vi "Get JSON Data.vi"(7 "Panel Origin":T1, 8 "error in (no error)":errorcluster, 9 "Force Get All Data":bool, 10 "VI Reference":refnum<vi>, 11 "Text In":refnum<class "Text.lvclass">) -> (0 "error out":errorcluster, 2 "JSON string":string, 3 "Text Out":refnum<class "Text.lvclass">)   [LabVIEW 2015, in "Front Panel Publisher.lvlib" / "Text.lvclass"]
uses:
  Text.lvclass
  <vilib>/Utility/miscctls.llb/LVPointTypeDef.ctl
  Object_class/Object.lvclass
  Web Front Panel_class/Web Front Panel.lvclass
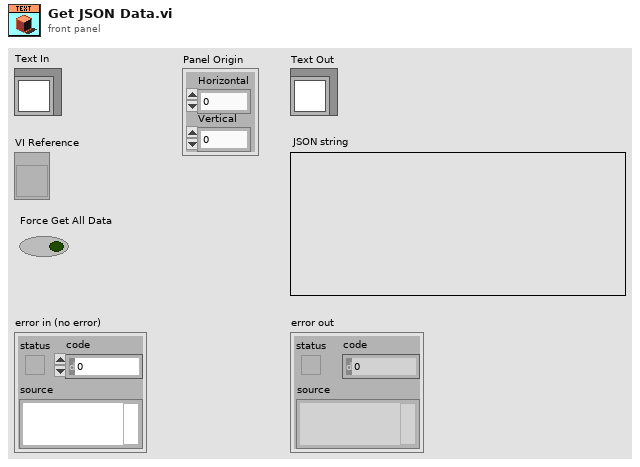
[diagram p1: front panel]
types:
  T1 = typedef "LVPointTypeDef.ctl" = cluster{"Horizontal":i16, "Vertical":i16}
  T2 = typedef "Front Panel Publisher.lvlib/Text.lvclass/Attributes.ctl" = cluster{"Text":string, "Font":string, "Font Size":u32, "Visible":bool, "Control Reference":refnum<vi>}
  T3 = typedef "Front Panel Publisher.lvlib/Object.lvclass/Attributes.ctl" = cluster{"UID":i32, "Type":string, "Coordinates":T4, "Reference":refnum<vi>}
  T4 = typedef "Front Panel Publisher.lvlib/Object.lvclass/Coordinates.ctl" = cluster{"Left":i32, "Top":i32, "Height":u32, "Width":u32}
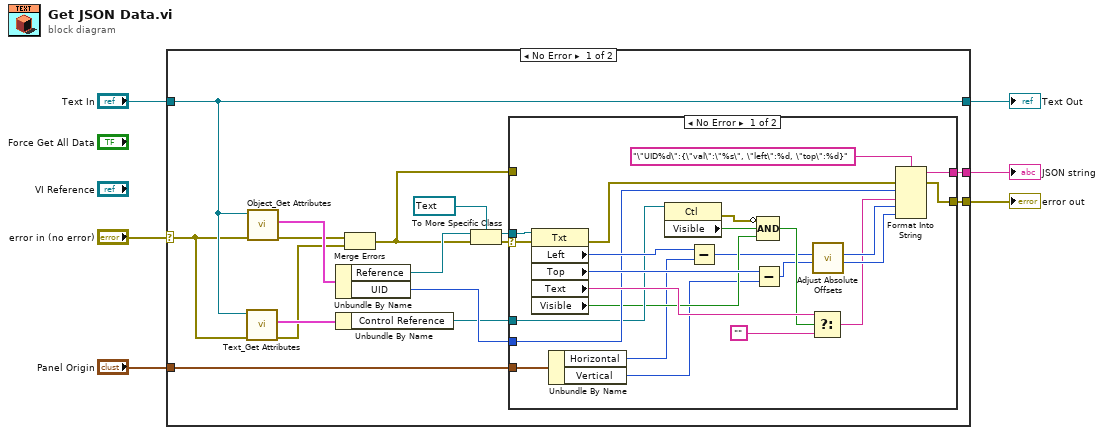
[diagram p0: block diagram]
diagram:
  n1 = case shown="No Error" "error in (no error)" {
    selector: "error in (no error)" -> [w8 w49]
    tunnel: [w21 _] -> w5
    tunnel: "Text In" -> [w13 w48]
    tunnel: [w20 w49] -> w3
    tunnel: [w13 w48] -> w2
    tunnel: "Panel Origin" -> [w7 _]
    frame No Error {
      n2 = call "Text_Get Attributes.vi"("error in (no error)"=w8, "Text In"=w13) -> ("error out"=w9:errorcluster, "Data"=w12:T2)  [unwired: 6 in, 2 out]
      n3 = call "Object_Get Attributes.vi"("error in (no error)"=w8, "Object In"=w13) -> ("error out"=w15:errorcluster, "Data"=w22:T3)  [unwired: 6 in, 2 out]
      n4 = Unbundle By Name(w22) -> ("Reference"=w14:refnum<vi>, "UID"=w16:i32)
      n5 = Unbundle By Name(w12) -> ("Control Reference"=w11:refnum<vi>)
      n6 = Merge Errors(w15, w9) -> (w10:errorcluster)
      n7 = To More Specific Class(target class=refnum<vi> refnum ("Caption"), reference=w14, error in=w10) -> (specific class reference=w18:refnum<vi>, error out=w19:errorcluster)
      n8 = case shown="No Error" w19 {
        selector: w19 -> [w39 _]
        tunnel: [w45 _] -> w21
        tunnel: [w40 w47] -> w20
        tunnel: w18 -> [w38 _]
        tunnel: w16 -> [w34 _]
        tunnel: w10 -> [_ w47]
        tunnel: w11 -> [w33 _]
        tunnel: w7 -> [w27 _]
        frame No Error {
          n9 = property class="Txt"(reference=w38, error in=w39) -> (error out=w41:errorcluster, "Left"=w44:i32, "Top"=w43:i32, "Text"=w36:string, "Visible"=w28:bool)  [unwired: 1 out]
          n10 = Unbundle By Name(w27) -> ("Horizontal"=w24:i16, "Vertical"=w23:i16)
          n11 = property class="Ctl"(reference=w33) -> (error out=w29:errorcluster, "Visible"=w32:bool)  [unwired: 1 in, 1 out]
          n12 = Subtract(x=w44, y=w24) -> (x-y=w26:i32)
          n13 = Subtract(x=w43, y=w23) -> (x-y=w25:i32)
          n14 = Compound Arithmetic op=AND(invert w29, w32, w28) -> (w30:bool)
          n15 = Select(t=w36, s=w30, f="") -> (s? t:f=w35:string)
          n16 = call "Adjust Absolute Offsets.vi"("Top In"=w25, "Left In"=w26) -> ("Top Out"=w42:i32, "Left Out"=w37:i32)  [unwired: 7 in, 1 out]
          n17 = Format Into String(format string="\"UID%d\":{\"val\":\"%s\", \"left\":%d, \"top\":%d}", error in=w41, w34, w35, w37, w42) -> (resulting string=w45:string, error out=w40:errorcluster)  [unwired: 1 in]
        }
        frame Error {
        }
      }
    }
    frame Error {
    }
  }
  "error out" <- w3
  "Text Out" <- w2
  "JSON string" <- w5
